vi "Event_CallBack.vi"(4 "Variant":variant, 5 "Event Data":cluster{"pDisp":variant, "URL":variant}, 6 "Control Ref":refnum<k7>, 7 "Event Common Data":T1) -> (1 "Event Data Out":cluster{"URL":variant})   [LabVIEW 2016, in "WebBrowser_Mgmt.lvclass"]
uses:
  WebBrowser_Mgmt.lvclass
  <vilib>/WebServerConfig/Action.ctl
  <vilib>/regexp/Match Regular Expression.xnode
  <userlib>/_OpenG.lib/file/file.llb/Strip Path Extension - String__ogtk.vi
panel:
  out "WebBrowser_Mgmt out":refnum<class "WebBrowser_Mgmt.lvclass">
  in  "WebBrowser_Mgmt in":refnum<class "WebBrowser_Mgmt.lvclass">
  out "error out":errorcluster
  in  "error in (no error)":errorcluster
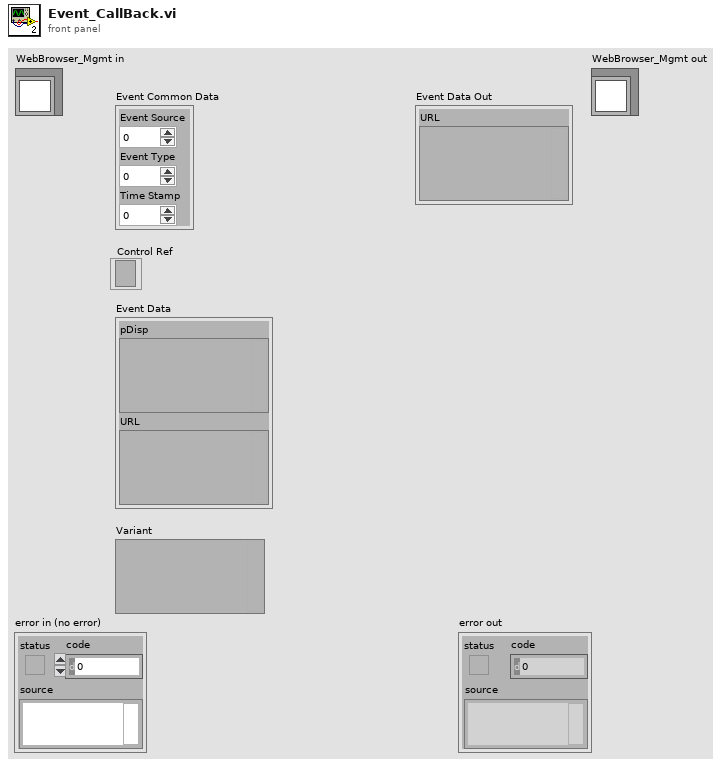
[diagram p1: front panel]
types:
  T1 = cluster{"Event Source":i32, "Event Type":u32, "Time Stamp":u32}
  T2 = typedef "Action.ctl" = enum16{"Nav Complete", "clicked PDF", "click Temp", "clicked SWF", "Not Valid"}
  T3 = typedef "Action.ctl" = cluster{"mimeType":string, "programPath":string}
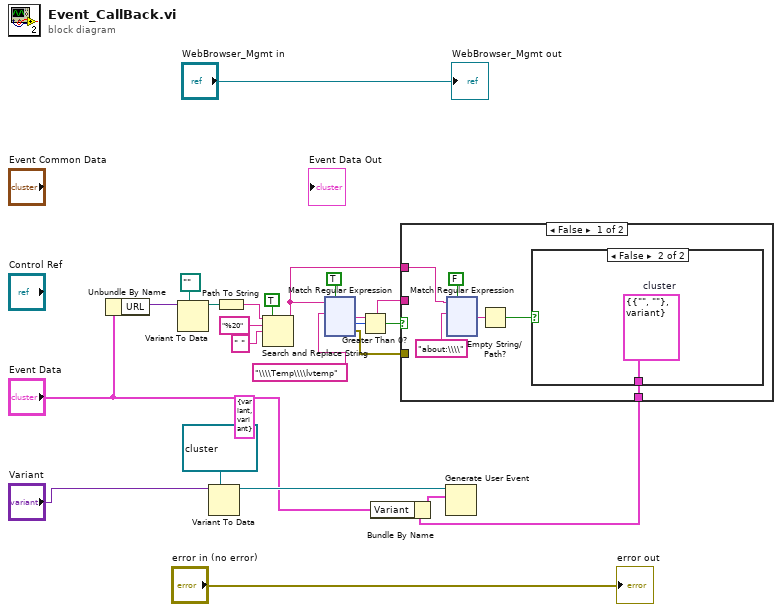
[diagram p0: block diagram]
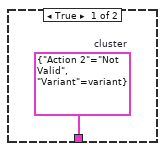
[diagram p2: hidden frame]
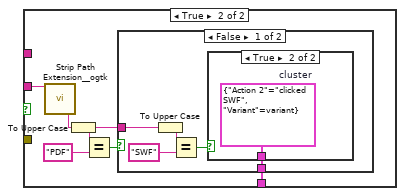
[diagram p3: hidden frame]
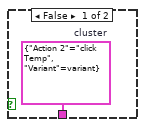
[diagram p4: hidden frame]
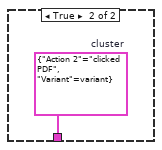
[diagram p5: hidden frame]
diagram:
  (unwired) cluster{"pDisp":variant, "URL":variant} {"pDisp"=variant, "URL"=variant} ("Event Data")
  n1 = Unbundle By Name("Event Data") -> ("URL"=w15:variant)
  n2 = Variant To Data(type=path "", Variant=w15) -> (data=w14:path)  [unwired: 1 in, 1 out]
  n3 = Variant To Data(type=refnum<user-event> refnum ("user event out"), Variant="Variant") -> (data=w20:refnum<user-event>)  [unwired: 1 in, 1 out]
  n4 = Path To String(path=w14) -> (string=w6:string)
  n5 = Search and Replace String(replace all?=TRUE ("replace all? (F)"), input string=w6, search string="%20", replace string=" " ("replace string (\"\")")) -> (result string=w1:string)  [unwired: 4 in, 3 out]
  n6 = xnode "Match Regular Expression"("input string"=w1, "regular expression"="\\\\Temp\\\\lvtemp", "ignore case? (F)"=TRUE) -> ("after match"=w2:string, "offset past match"=w7:i32, "error out"=w4:errorcluster)  [unwired: 3 in, 2 out]
  n7 = Greater Than 0?(x=w7) -> (x > 0?=w5:bool)
  n8 = case shown="False" w5 {
    tunnel: [w28 w147] -> w10
    tunnel: w4 -> [_ _]
    tunnel: w2 -> [_ w146]
    tunnel: w1 -> [w25 _]
    frame False {
      n9 = xnode "Match Regular Expression"("input string"=w25, "regular expression"="about:\\\\", "ignore case? (F)"=FALSE) -> ("after match"=w24:string)  [unwired: 3 in, 4 out]
      n10 = Empty String/Path?(string/path=w24) -> (empty?=w23:bool)
      n11 = case shown="False" w23 {
        tunnel: [w29 w30] -> w28
        frame True {
          w29 = cluster{"Action 2":T2, "Variant":variant} {"Action 2"=enum."Not Valid", "Variant"=variant}  # cluster
        }
        frame False {
          w30 = cluster{"Action 2":T3, "Variant":variant} {"Action 2"={"mimeType"="", "programPath"=""}, "Variant"=variant}  # cluster
        }
      }
    }
    frame True {
      n12 = call-poly <userlib>:"Strip Path Extension__ogtk.vi"("path"=w146) -> ("extension"=w150:string)  [unwired: 1 out]
      n13 = To Upper Case(1:w150) -> (0:w145:string)
      n14 = Equal?(x=w145, y="PDF") -> (x = y?=w148:bool)
      n15 = case shown="False" w148 {
        tunnel: [w155 w158] -> w147
        tunnel: w145 -> [w152 _]
        frame False {
          n16 = To Upper Case(1:w152) -> (0:w153:string)
          n17 = Equal?(x=w153, y="SWF") -> (x = y?=w151:bool)
          n18 = case shown="True" w151 {
            tunnel: [w156 w157] -> w155
            frame False {
              w156 = cluster{"Action 2":T2, "Variant":variant} {"Action 2"=enum."click Temp", "Variant"=variant}  # cluster
            }
            frame True {
              w157 = cluster{"Action 2":T2, "Variant":variant} {"Action 2"=enum."clicked SWF", "Variant"=variant}  # cluster
            }
          }
        }
        frame True {
          w158 = cluster{"Action 2":T2, "Variant":variant} {"Action 2"=enum."clicked PDF", "Variant"=variant}  # cluster
        }
      }
    }
  }
  n19 = Bundle By Name(cluster=w10, "Variant"="Event Data") -> (w3:cluster{"Action 2":T3, "Variant":variant})
  n20 = Generate User Event(user event=w20, event data cluster=w3) -> ()  [unwired: 2 in, 2 out]
  "error out" <- "error in (no error)"
  "WebBrowser_Mgmt out" <- "WebBrowser_Mgmt in"
